vi "ArdnoManualValves.vi"() -> ()   [LabVIEW 2018]
uses:
  <vilib>/MakerHub/LINX/Public/Peripherals/Digital/Digital Write N Chans.vi
  <vilib>/MakerHub/LINX/Private/Local IO/LinxDigitalWrite.vi
  <vilib>/MakerHub/LINX/Public/Utilities/Check Channel.vi
  <vilib>/MakerHub/LINX/Public/Utilities/Open Serial.vi
  <vilib>/MakerHub/LINX/Private/Utilties/Generate Error.vi
  <vilib>/MakerHub/LINX/LMH-LINX.lvlib
panel:
  out "Error Out":errorcluster
  out "Device Name":string
  in  "error in (no error)":errorcluster
  in  "VISA resource name":refnum<visa-resource-name>
  in  "Manually controlled Valves":u8[](array[numeric])
  out "Open?":bool
  in  "Manual Open":bool
  in  "stop":bool
  # "ALWAYS TERMINATE THE\nPROGRAM WITH THIS STOP BUTTON!"
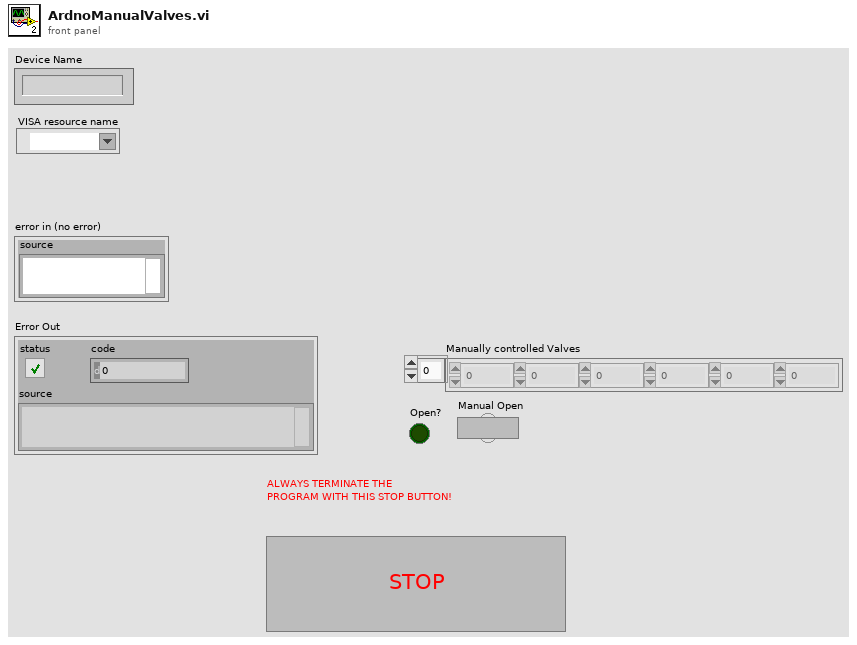
[diagram p1: front panel]
types:
  T1 = typedef "LMH-LINX.lvlib/LINX Ref.ctl" = cluster{"IO":T2, "Interface":T3, "LINX Device Config":T4}
  T2 = typedef "LMH-LINX.lvlib/Platform.ctl" = enum16{"Remote", "Local"}
  T3 = typedef "LMH-LINX.lvlib/Interface.ctl" = enum16{"Serial", "TCP"}
  T4 = typedef "LMH-LINX.lvlib/Device.lvlib/LINX Device Config.ctl" = cluster{"Interface":T3, "COM Port":refnum<visa-resource-name>, "TCP Configuration":T5, "Device Family":u8, "Device ID":u8, "Device Name":string, "TCP Ref":refnum<k5>, "Channels":T6}
  T5 = typedef "LMH-LINX.lvlib/Device.lvlib/TCP Config.ctl" = cluster{"IP Address":string, "Port":u16}
  T6 = typedef "LMH-LINX.lvlib/Channels.ctl" = cluster{"DI":u8[], "DO":u8[], "AI":u8[], "AO":u8[], "PWM":u8[], "QE":u8[], "UART":u8[], "I2C 2":u8[], "SPI":u8[], "CAN":u8[], "Servo":u8[], "AI Ref (V)":dbl, "AI Resolution (Bits)":u8, "AO Ref (V)":dbl, "AO Resolution (Bits)":u8}
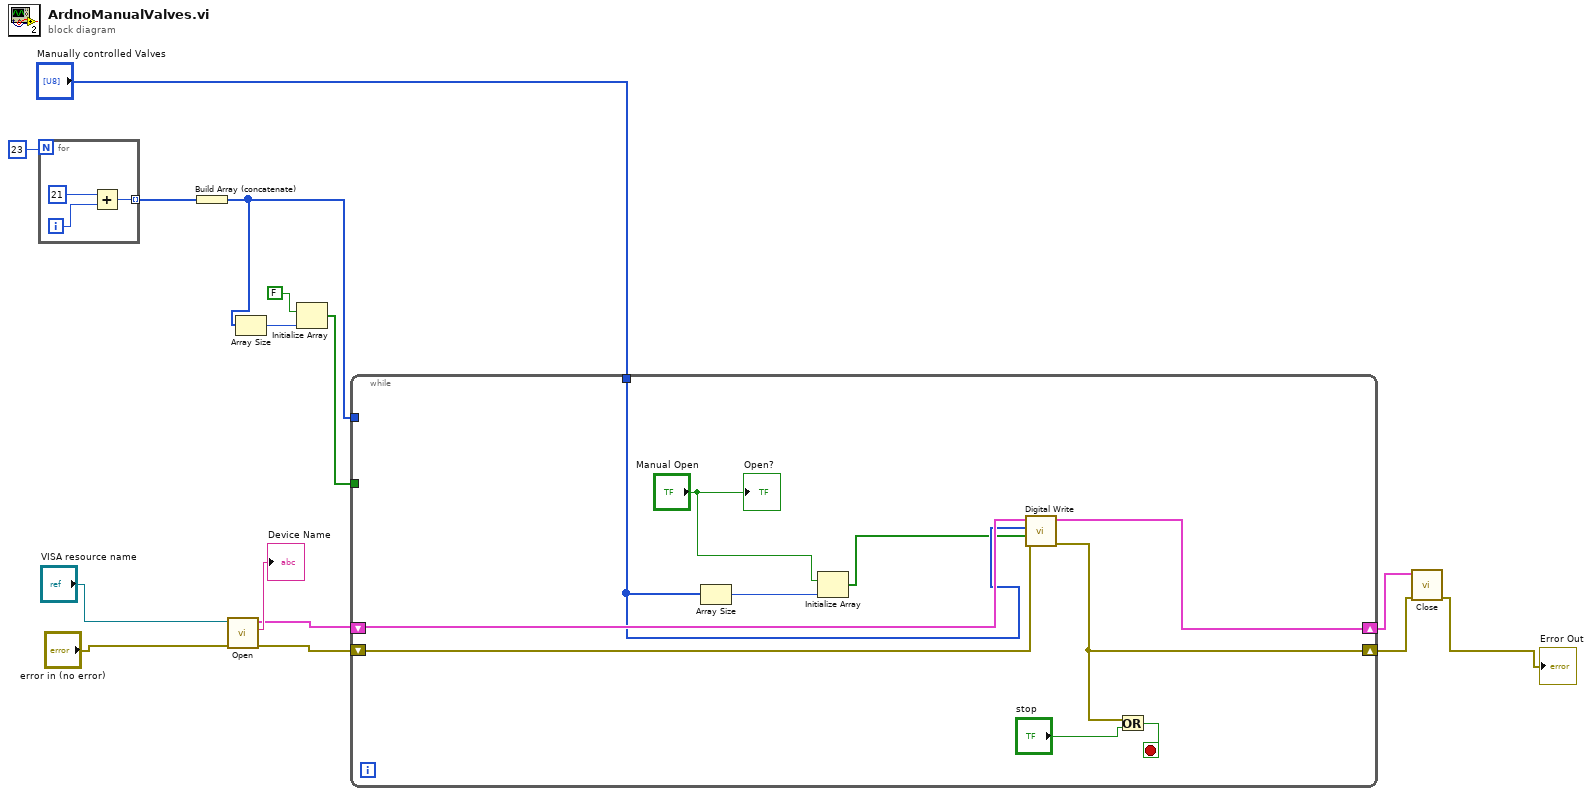
[diagram p0: block diagram]
diagram:
  n1 = for {
    N: 23 -> [_]
    tunnel: [w16] -> w14 mode=indexing
    i -> [w18]
    n2 = Add(x=21, y=w18) -> (x+y=w16:i32)
  }
  n3 = Build Array (concatenate)(w14) -> (w13:i32[])
  n4 = call-poly <vilib>:"Open.vi"("Error In"="error in (no error)", "Serial Port"="VISA resource name") -> ("Error Out"=w3:errorcluster, "Device Name"=→"Device Name":string, "LINX Resource"=w1:T1)  [unwired: 7 in]
  n5 = Array Size(array=w13) -> (size(s)=w12:i32)
  n6 = Initialize Array(FALSE, w12) -> (w10:bool[])
  n7 = while {
    tunnel: w13 -> [_]
    tunnel: w10 -> [_]
    tunnel: "Manually controlled Valves" -> [w23]
    shift-right: [w19] -> w8
    shift-left: w1 -> [w24]
    shift-right: [w20] -> w7
    shift-left: w3 -> [w21]
    stop <- w27 stop-if-true
    n8 = Array Size(array=w23) -> (size(s)=w26:i32)
    n9 = Initialize Array("Manual Open", w26) -> (w22:bool[])
    n10 = call-poly <vilib>:"Digital Write.vi"("Error In"=w21, "Values"=w22, "DO Channels"=w23, "LINX Resource"=w24) -> ("Error Out"=w20:errorcluster, "LINX Resource"=w19:T1)  [unwired: 6 in]
    n11 = Or(x=w20, y="stop") -> (x .or. y?=w27:bool)
    "Open?" <- "Manual Open"
  }
  n12 = call <vilib>:"Close.vi"("Error In"=w7, "LINX Resource"=w8) -> ("Error Out"=→"Error Out":errorcluster)  [unwired: 9 in]
